vi "Unflatten XML.vi"(8 "Error In":errorcluster, 10 "XML":string, 11 "UIM In":refnum<data-value>) -> (0 "Error Out":errorcluster, 3 "UIM Out":refnum<data-value>)   [LabVIEW 2020, in "UIM.lvlib" / "UIM.lvclass"]
doc: "This method will convert the UIM data from XML format that is easy to read. The same format is used when the UIM is saved and loaded to and from XML file.\n\n<b>Important </b>- If the XML specifies the <UIPList> only the plugins specified in that list will be used and loaded with the file. Make sure that the list specifies ALL the plugins used in the UIM States. Otherwise they will not be loaded. If the <UIPList> is not present in the file then the default UIPs and the UIPs from the Plugin folder will be used."
uses:
  UIM.lvclass
  <vilib>/xml/Close Reference(Node).vi
  UIM.lvclass/UIM.ctl
  <vilib>/xml/NI_XML.lvlib
  <resource>/objmgr/DOMUserDefRef.rc
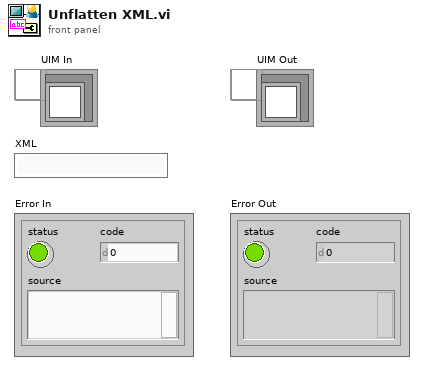
[diagram p1: front panel]
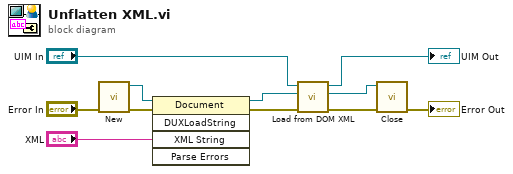
[diagram p0: block diagram]
diagram:
  n1 = call <vilib>:"New.vi"("error in (no error)"="Error In") -> ("error out"=w10:errorcluster, "DOM document out"=w11:refnum<k20>)  [unwired: 7 in]
  n2 = invoke class="Document" method="DUXLoadString"(reference=w11, error in=w10, "XML String"="XML") -> (reference out=w4:refnum<k20>, error out=w6:errorcluster)  [unwired: 2 in, 3 out]
  n3 = call "Load from DOM XML.vi"("Error In"=w6, "DOM In"=w4, "UIM In"="UIM In") -> ("Error Out"=w5:errorcluster, "DOM Out"=w3:refnum<k20>, "UIM Out"=→"UIM Out":refnum<data-value>)  [unwired: 6 in]
  n4 = call-poly <vilib>:"Close.vi"("error in (no error)"=w5, "node"=w3) -> ("error out"=→"Error Out":errorcluster)  [unwired: 7 in]
